vi "CVT2TagNotFoundTest.vi"() -> (3 "Unit Test Framework Results":T1)   [LabVIEW 2013, in "UnitTests.lvlib"]
uses:
  UnitTests.lvlib
  <vilib>/utf/common/utf_test_result_troll.ctl
  <vilib>/utf/common/utf_test_result.ctl
  <vilib>/utf/common/utf_test_result_failure.ctl
  <vilib>/utf/common/utf_test_comparison_operators.ctl
  <vilib>/utf/common/utf_vi_tag.ctl
  <vilib>/NI/Current Value Table/DataTypes/I32_Read.vi
  <vilib>/NI/Current Value Table/Type to Enum.vi
  <vilib>/NI/Current Value Table/DataTypes/I32_Type To Enum.vi
  <vilib>/NI/Current Value Table/FGVs/CVT Globals.vi
  <vilib>/NI/Current Value Table/FGVs/Tag Memory.vi
  <vilib>/NI/Current Value Table/Memory Block.vi
  <vilib>/NI/Current Value Table/DataTypes/I32_Memory Block.vi
  <vilib>/utf/NI_UnitTestFramework.lvlib
  <vilib>/NI/Current Value Table/Current Value Table.lvlib
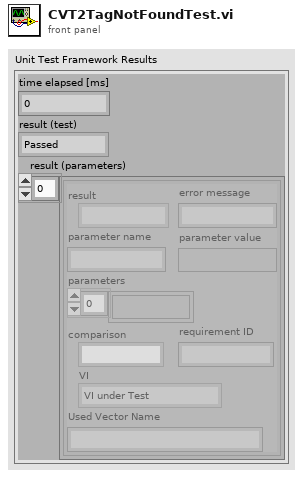
[diagram p1: front panel]
types:
  T1 = typedef "NI_UnitTestFramework.lvlib/utf_test_result_troll.ctl" = cluster{"time elapsed [ms]":u32, "result (test)":T2, "result (parameters)":T3[]}
  T2 = typedef "NI_UnitTestFramework.lvlib/utf_test_result.ctl" = enum16{"Passed", "Failed", "Error", "Skipped", "Not Processed"}
  T3 = typedef "NI_UnitTestFramework.lvlib/utf_test_result_failure.ctl" = cluster{"result":T2, "error message":string, "parameter name":string, "parameter value":variant, "parameters":variant[], "comparison":T4, "requirement ID":string, "VI":T5, "Used Vector Name":string}
  T4 = typedef "NI_UnitTestFramework.lvlib/utf_test_comparison_operators.ctl" = enum16{"=", "!=", ">", ">=", "<", "<=", "range", "symmetric tolerance", "asymmetric tolerance", "string contains", "string not contain", "array size", "string length", "array range", "by element", "array range (limit array)", "user-defined", "array contains", "array not contain", "vector length", "= (elm)", "!= (elm)", "= (case insensitive)", "!= (case insensitive)"}
  T5 = typedef "NI_UnitTestFramework.lvlib/utf_vi_tag.ctl" = enum16{"Setup VI", "VI under Test", "Teardown VI"}
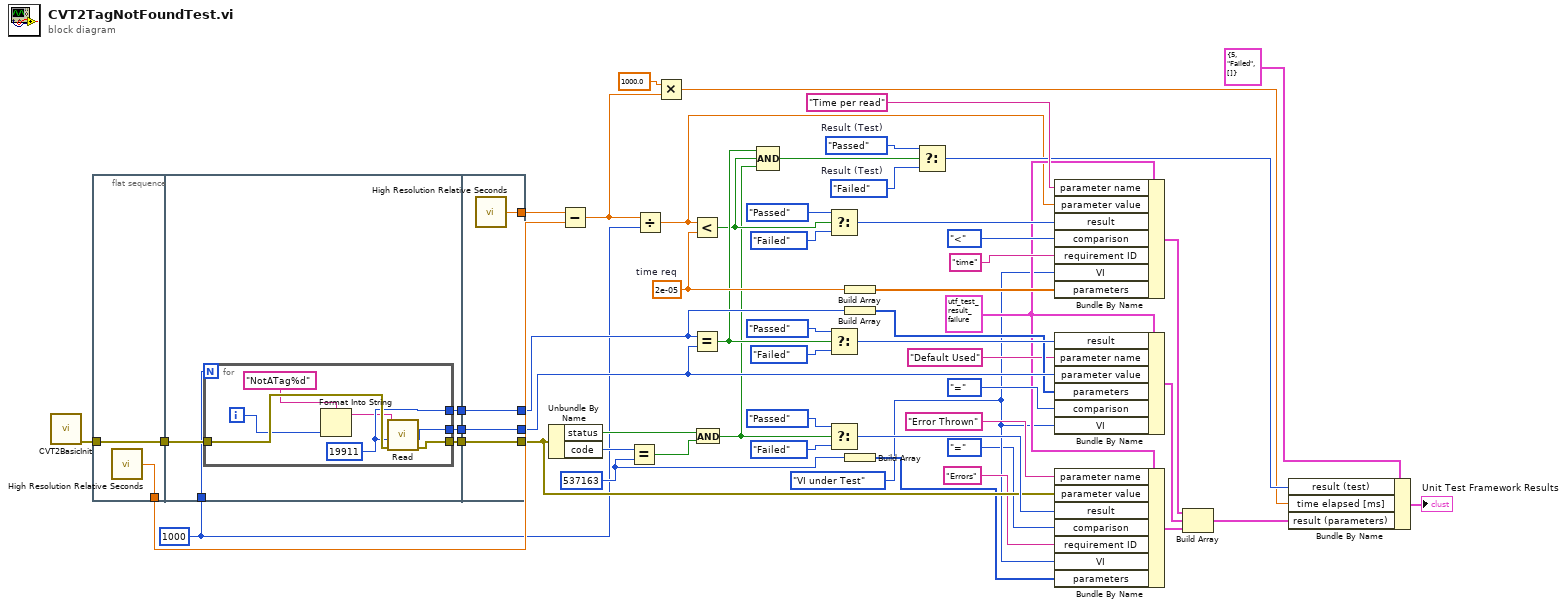
[diagram p0: block diagram]
diagram:
  w2 = 1000
  w15 = utf_test_result."Passed"  # Result (Test)
  w16 = utf_test_result."Failed"  # Result (Test)
  w7 = 537163 ("y")
  w5 = utf_vi_tag."VI under Test" ("VI")
  w39 = 2e-05  # time req
  w29 = T3 {"result"=enum."Passed", "error message"="", "parameter name"="", "parameter value"=variant, "parameters"=[], "comparison"=enum."=", "requirement ID"="", "VI"=enum."Setup VI", "Used Vector Name"=""} ("Unit Test Framework - result (parameters)")
  n1 = call "CVT2BasicInit.vi"() -> ("error out"=w51:errorcluster)  [unwired: 9 in, 2 out]
  n2 = flat-sequence {
    tunnel: [w57] -> w52
    tunnel: w51 -> [w56]
    tunnel: [w56] -> w50
    tunnel: w50 -> [w62]
    tunnel: [w61] -> w49
    tunnel: [w60] -> w48
    tunnel: [w59] -> w47
    tunnel: w2 -> [w58]
    tunnel: [w73] -> w53
    tunnel: [w72] -> w9
    tunnel: w49 -> [w72]
    tunnel: [w71] -> w35
    tunnel: w48 -> [w71]
    tunnel: w47 -> [w70]
    tunnel: [w70] -> w33
    frame #0 {
      n3 = call <vilib>:"High Resolution Relative Seconds.vi"() -> ("relative seconds"=w57:dbl)
    }
    frame #1 {
      n4 = for {
        N: w58 -> [_]
        tunnel: [w69] -> w60
        tunnel: [w66] -> w59
        tunnel: w62 -> [w68]
        tunnel: [w67] -> w61
        i -> [w65]
        w66 = 19911 ("Default")
        n5 = Format Into String(format string="NotATag%d" ("Tag Name"), w65) -> (resulting string=w63:string)  [unwired: 2 in, 1 out]
        n6 = call-poly <vilib>:"Read.vi"("error in (no error)"=w68, "Default"=w66, "Tag Name"=w63) -> ("error out"=w67:errorcluster, "Value"=w69:i32)  [unwired: 7 in]
      }
    }
    frame #2 {
      n7 = call <vilib>:"High Resolution Relative Seconds.vi"() -> ("relative seconds"=w73:dbl)
    }
  }
  n8 = Unbundle By Name(w9) -> ("status"=w22:bool, "code"=w24:i32)
  n9 = Subtract(x=w53, y=w52) -> (x-y=w3:dbl)
  n10 = Equal?(x=w24, y=w7) -> (x = y?=w23:bool)
  n11 = Divide(x=w3, y=w2) -> (x/y=w1:dbl)
  n12 = Multiply(x=1000.0 ("y"), y=w3) -> (x*y=w12:dbl)
  n13 = Less?(x=w1, y=w39) -> (x < y?=w18:bool)
  n14 = Equal?(x=w33, y=w35) -> (x = y?=w19:bool)
  n15 = And(x=w22, y=w23) -> (x .and. y?=w17:bool)
  n16 = Compound Arithmetic op=AND(w19, w18, w17) -> (w14:bool)
  n17 = Select(t=utf_test_result."Passed" ("result"), s=w18, f=utf_test_result."Failed" ("result")) -> (s? t:f=w41:T2)
  n18 = Select(t=utf_test_result."Passed" ("result"), s=w19, f=utf_test_result."Failed" ("result")) -> (s? t:f=w36:T2)
  n19 = Select(t=utf_test_result."Passed" ("result"), s=w17, f=utf_test_result."Failed" ("result")) -> (s? t:f=w10:T2)
  n20 = Build Array(w39) -> (w40:dbl[])
  n21 = Build Array(w33) -> (w34:i32[])
  n22 = Build Array(w7) -> (w8:i32[])
  n23 = Select(t=w15, s=w14, f=w16) -> (s? t:f=w13:T2)
  n24 = Bundle By Name(cluster=w29, "parameter name"="Time per read", "parameter value"=w1, "result"=w41, "comparison"=utf_test_comparison_operators."<", "requirement ID"="time", "VI"=w5, "parameters"=w40) -> (w28:T3)
  n25 = Bundle By Name(cluster=w29, "result"=w36, "parameter name"="Default Used", "parameter value"=w35, "parameters"=w34, "comparison"=utf_test_comparison_operators."=", "VI"=w5) -> (w27:T3)
  n26 = Bundle By Name(cluster=w29, "parameter name"="Error Thrown", "parameter value"=w9, "result"=w10, "comparison"=utf_test_comparison_operators."=", "requirement ID"="Errors" ("parameter name"), "VI"=w5, "parameters"=w8) -> (w26:T3)
  n27 = Build Array(w28, w27, w26) -> (w11:T3[])
  n28 = Bundle By Name(cluster=T1 {"time elapsed [ms]"=5, "result (test)"=enum."Failed", "result (parameters)"=[]} ("Unit Test Framework - Result"), "result (test)"=w13, "time elapsed [ms]"=w12, "result (parameters)"=w11) -> (→"Unit Test Framework Results":T1)
